vi "kSAComm Text Command.vi"(0 "kSAComm Ref In":refnum<k24>, 1 "Command":string) -> (2 "kSAComm Ref Out":refnum<k24>, 3 "Status":i32(ring) items=["ERR_SUCCESS"=0, "ERR_CONNECTION"=-5, "ERR_STATE"=-4, "ERR_PARAM"=-3, "ERR_UNKOWN"=-2, "ERR_GENERAL"=-1], 4 "Response":string)   [LabVIEW 2019]
uses:
  C:/Users/tim/Documents/kSAComm LabView Sample/kSACommInterface.dll
  kSACommInterface.dll
panel:
  in  "IP":string="192.168.0.169"
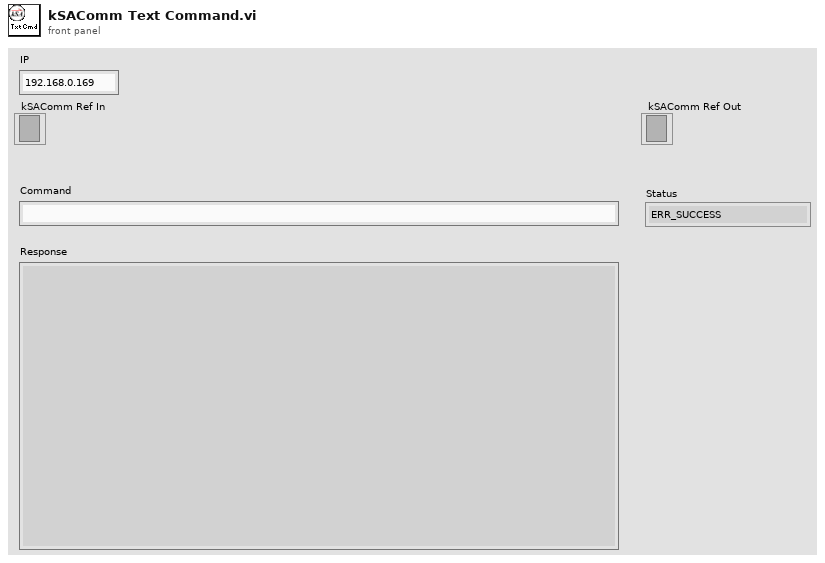
[diagram p1: front panel]
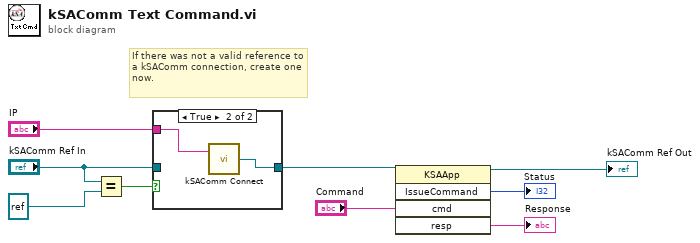
[diagram p0: block diagram]
diagram:
  # "If there was not a valid reference to a kSAComm connection, create one now."
  n1 = Equal?(x="kSAComm Ref In", y=refnum<k24> refnum ("kSAComm Ref")) -> (x = y?=w5:bool)
  n2 = case shown="True" w5 {
    tunnel: "kSAComm Ref In" -> [w10 _]
    tunnel: [w10 w12] -> w3
    tunnel: "IP" -> [_ w11]
    frame False {
    }
    frame True {
      n3 = call "kSAComm Connect.vi"("IP Address"=w11) -> ("kSAComm ref out"=w12:refnum<k24>)  [unwired: 2 in, 1 out]
    }
  }
  n4 = invoke class="KSAApp" method="IssueCommand"(reference=w3, "cmd"="Command") -> (reference out=→"kSAComm Ref Out":refnum<k24>, "IssueCommand"=→"Status":i32, "resp"=→"Response":string)  [unwired: 3 in, 2 out]
